vi "NicmosStop.vi"(9 "error in (no error)":errorcluster caption="error out (no error)") -> (6 "error out":errorcluster)   [LabVIEW 2009]
uses:
  Controls/NICMOS.STATE.ctl
  Controls/NICMOS.COMMAND.ctl
  Controls/NICMOS.COMMANDBASIC.ctl
  Controls/NICMOS.READOUT.ctl
  Controls/NICMOS.FILTERCOMMAND.ctl
  Controls/NICMOS.FILTER.ctl
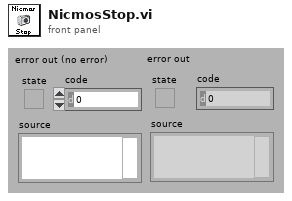
[diagram p1: front panel]
types:
  T1 = typedef "NICMOS.STATE.ctl" = enum16{"IDLE", "WRITING BANKS", "SETTING FILTER", "HOMING FILTER", "QUERYING TEMP", "CONFIGURING", "STARTING", "RUNNING", "HALTING", "STOPPED"}
  T2 = typedef "NICMOS.COMMAND.ctl" = cluster{"Command":T3, "READOUT":T4, "FILTERCOMMAND":T5, "ACQUISITION":i32, "Done":refnum<k4>}
  T3 = typedef "NICMOS.COMMANDBASIC.ctl" = enum16{"WRITE BANKS", "SET FILTER", "HOME FILTER", "QUERY TEMP", "CONFIGURE", "START", "ACQUISITION", "STOP", "QUIT"}
  T4 = typedef "NICMOS.READOUT.ctl" = cluster{"Readout":i32, "Deglitch":i32, "Framerate":dbl[unit], "Bank":i32}
  T5 = typedef "NICMOS.FILTERCOMMAND.ctl" = cluster{"FILTER":T6, "INIT":bool}
  T6 = typedef "NICMOS.FILTER.ctl" = string
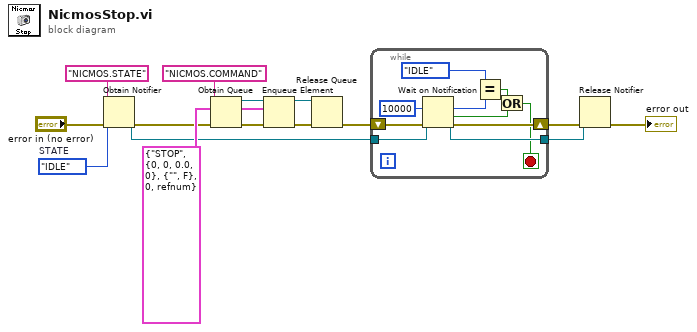
[diagram p0: block diagram]
diagram:
  w8 = NICMOS.STATE."IDLE"  # STATE
  w10 = T2 {"Command"=enum."STOP", "READOUT"={"Readout"=0, "Deglitch"=0, "Framerate"=0.0, "Bank"=0}, "FILTERCOMMAND"={"FILTER"="", "INIT"=FALSE}, "ACQUISITION"=0, "Done"=refnum} ("NicmosCommand")
  n1 = Obtain Notifier(name (unnamed)="NICMOS.STATE", notification data type=w8, error in (no error)="error in (no error)") -> (notifier out=w4:refnum<notifier>, error out=w6:errorcluster)  [unwired: 1 in, 1 out]
  n2 = Obtain Queue(name (unnamed)="NICMOS.COMMAND" ("nom (aucun)"), element data type=w10, error in (no error)=w6) -> (queue out=w12:refnum<queue>, error out=w15:errorcluster)  [unwired: 2 in, 1 out]
  n3 = Enqueue Element(queue=w12, element=w10, error in (no error)=w15) -> (queue out=w11:refnum<queue>, error out=w14:errorcluster)  [unwired: 1 in, 1 out]
  n4 = Release Queue(queue=w11, error in (no error)=w14) -> (error out=w5:errorcluster)  [unwired: 1 in, 2 out]
  n5 = while {
    tunnel: w4 -> [w23]
    shift-right: [w24] -> w3
    shift-left: w5 -> [w25]
    tunnel: [w22] -> w1
    stop <- w16 stop-if-true
    n6 = Wait on Notification(notifier=w23, timeout in ms (-1)=10000 ("timeout en ms (-1)"), error in (no error)=w25) -> (notifier out=w22:refnum<notifier>, notification=w20:T1, timed out?=w17:bool, error out=w24:errorcluster)  [unwired: 1 in]
    n7 = Equal?(x=NICMOS.STATE."IDLE" ("notification"), y=w20) -> (x = y?=w18:bool)
    n8 = Or(x=w18, y=w17) -> (x .or. y?=w16:bool)
  }
  n9 = Release Notifier(notifier=w1, error in (no error)=w3) -> (error out=→"error out":errorcluster)  [unwired: 1 in, 2 out]
